vi "Set Columns.vi"(3 "error in (no error)":errorcluster, 4 "Columns in":refnum<class "Column.lvclass">[](array[class]), 5 "Novatech in":refnum<class "Novatech.lvclass">) -> (0 "error out":errorcluster, 1 "Novatech out":refnum<class "Novatech.lvclass">)   [LabVIEW 2013, in "Novatech.lvclass"]
uses:
  Novatech.lvclass
  ColumnVIs/Column/Column.lvclass
  <vilib>/Utility/error.llb/DialogType.ctl
  Device/Device.lvclass
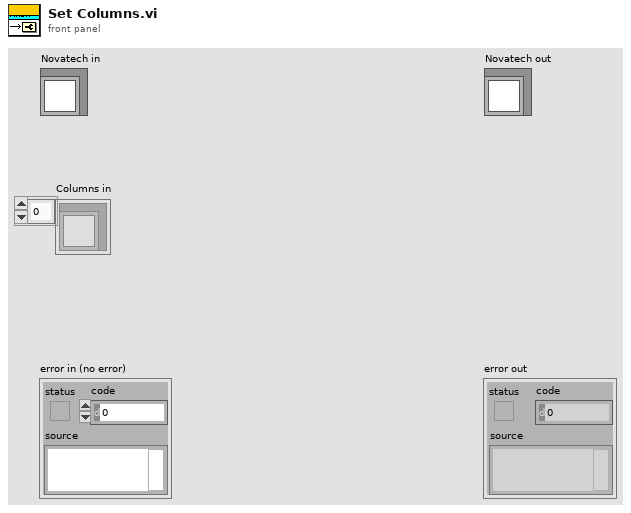
[diagram p1: front panel]
types:
  T1 = typedef "DialogType.ctl" = u16
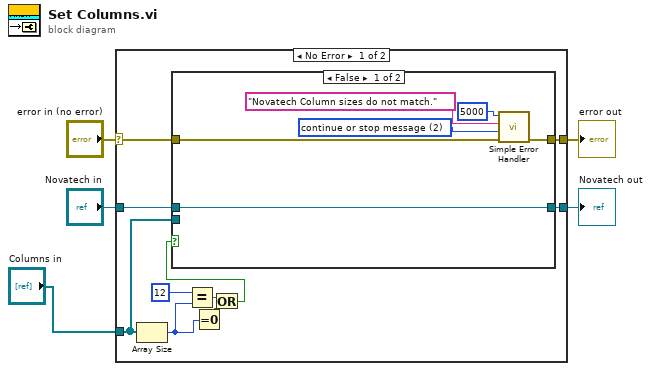
[diagram p0: block diagram]
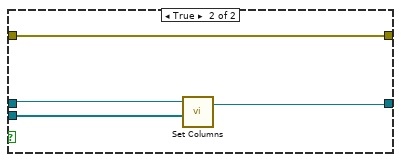
[diagram p2: hidden frame]
diagram:
  n1 = case shown="No Error" "error in (no error)" {
    selector: "error in (no error)" -> [w14 w26]
    tunnel: [w13 w26] -> w2
    tunnel: "Novatech in" -> [w12 w27]
    tunnel: "Columns in" -> [w11 _]
    tunnel: [w15 w27] -> w3
    frame No Error {
      n2 = Array Size(array=w11) -> (size(s)=w6:i32)
      n3 = Equal?(x=12 ("y"), y=w6) -> (x = y?=w10:bool)
      n4 = Equal To 0?(x=w6) -> (x = 0?=w8:bool)
      n5 = Or(x=w10, y=w8) -> (x .or. y?=w9:bool)
      n6 = case shown="False" w9 {
        tunnel: w12 -> [w21 w24]
        tunnel: w11 -> [_ w22]
        tunnel: [w21 w23] -> w15
        tunnel: w14 -> [w20 w25]
        tunnel: [w19 w25] -> w13
        frame False {
          w17 = T1 2 items=["no dialog", "OK message", "continue or stop message", "OK message + warnings", "continue/stop + warnings"] ("type of dialog (OK msg:1)")
          n7 = call <vilib>:"Simple Error Handler.vi"("error code (no error:0)"=5000, "error source (\" \")"="Novatech Column sizes do not match." ("message"), "type of dialog (OK msg:1)"=w17, "error in (no error)"=w20) -> ("error out"=w19:errorcluster)  [unwired: 1 in, 4 out]
        }
        frame True {
          n8 = call-parent "Set Columns.vi"("Columns"=w22, "Device in"=w24) -> ("Device out"=w23:refnum<class "Novatech.lvclass">)  [unwired: 2 in, 1 out]
        }
      }
    }
    frame Error {
    }
  }
  "error out" <- w2
  "Novatech out" <- w3
